vi "Convert_ERDS_GEA_Version.vi"(0 "New Header?":bool=TRUE, 2 "ERD Name":string[](array[string]), 5 "ERD_Data_Bound":T1, 7 "Multiple Read":T2 {"ERD Number" format="%x"}, 11 "error IO":errorcluster) -> (6 "All_ERD_Data_Bundled_Brass":T1, 15 "error out":errorcluster)   [LabVIEW 2021]
uses:
  Controles/Multiple_Read_ERD.ctl
  Controles/Read_ERD.ctl
  Controles/ERD_Data_Boundled.ctl
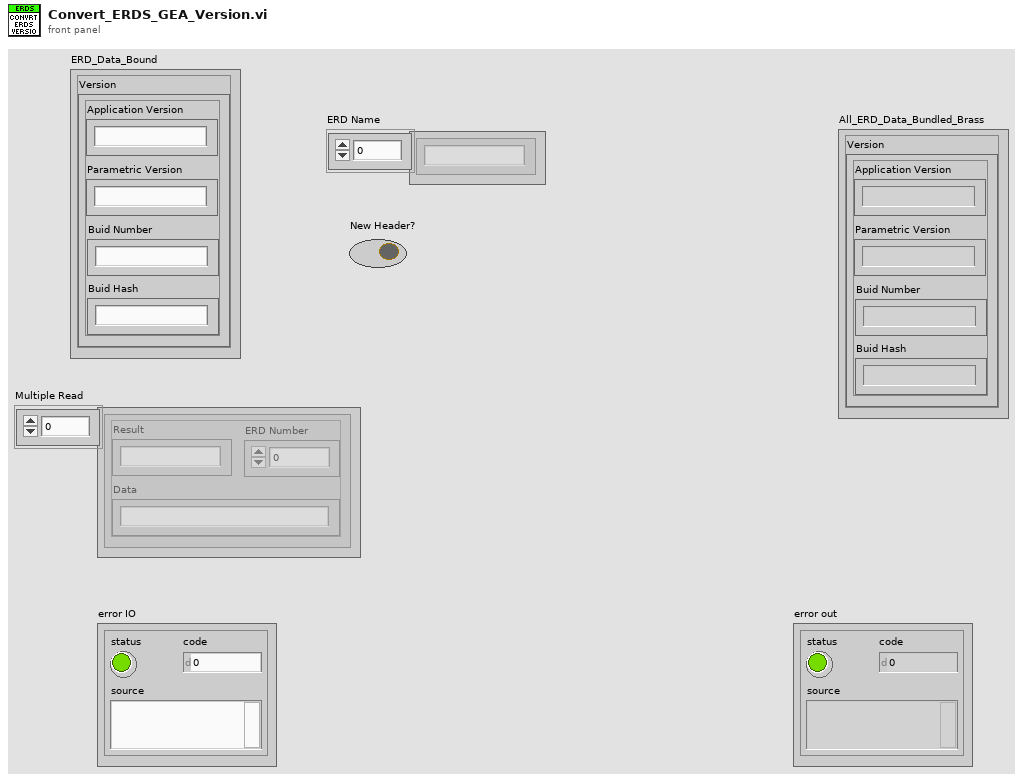
[diagram p1: front panel]
types:
  T1 = typedef "ERD_Data_Boundled.ctl" = cluster{"Version":cluster{"Application Version":string, "Parametric Version":string, "Buid Number":string, "Buid Hash":string}}
  T2 = typedef "Multiple_Read_ERD.ctl" = T3[]
  T3 = typedef "Read_ERD.ctl" = cluster{"Result":string, "ERD Number":i64, "Data":string}
  T4 = cluster{"Application Version":string, "Parametric Version":string, "Buid Number":string, "Buid Hash":string}
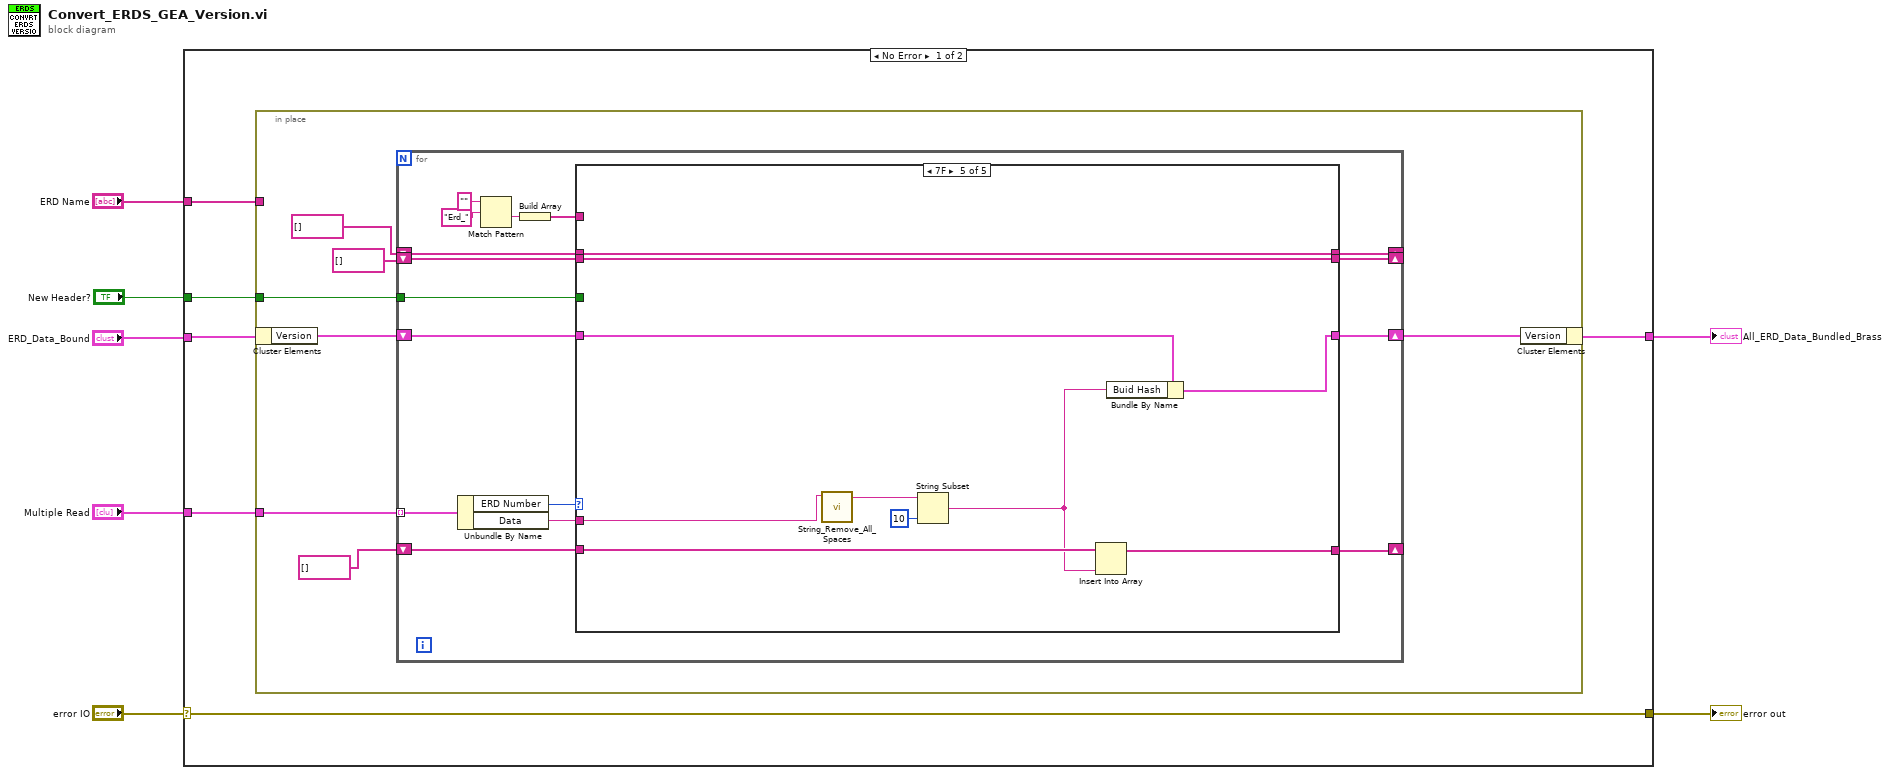
[diagram p0: block diagram]
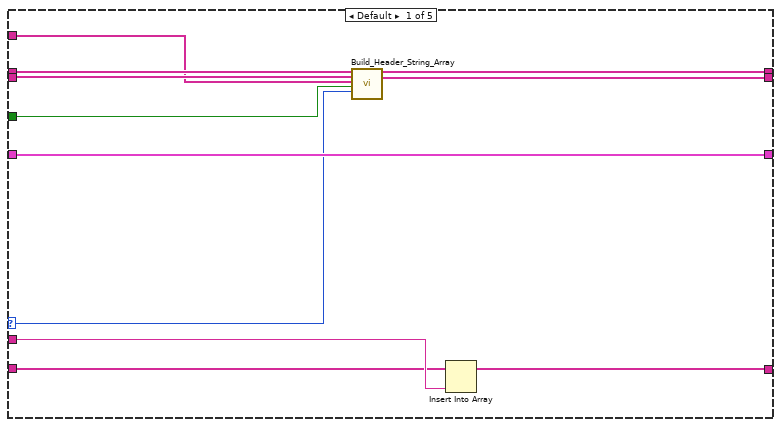
[diagram p2: hidden frame]
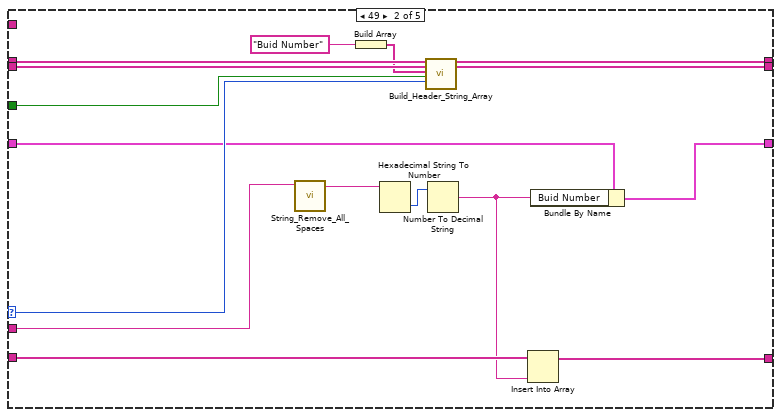
[diagram p3: hidden frame]
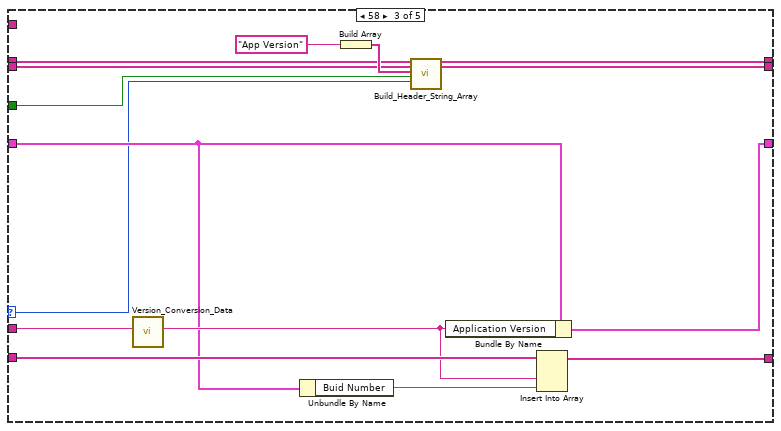
[diagram p4: hidden frame]
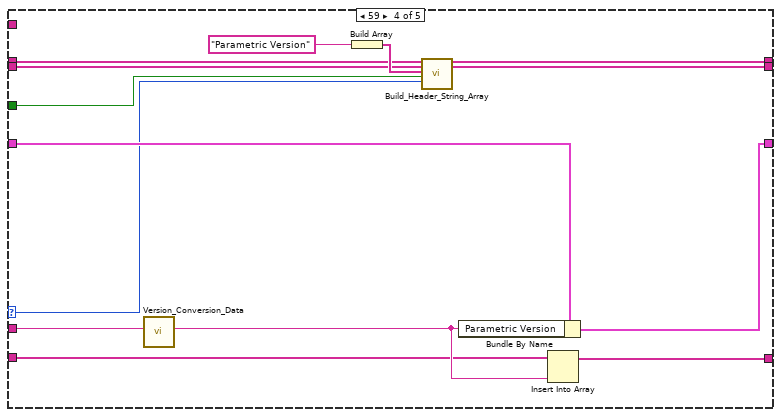
[diagram p5: hidden frame]
diagram:
  n1 = case shown="No Error" "error IO" {
    selector: "error IO" -> [w9 w103]
    tunnel: "ERD_Data_Bound" -> [w13 _]
    tunnel: "Multiple Read" -> [w12 _]
    tunnel: "ERD Name" -> [w11 _]
    tunnel: "New Header?" -> [w10 _]
    tunnel: [w9 w103] -> w2
    tunnel: [w8 _] -> w1
    frame No Error {
      n2 = in-place {
        in-place-border: w12 -> [w20]
        in-place-border: w11 -> [_]
        in-place-border: w10 -> [w15]
        n3 = in-place-cluster #1(w13) -> ("Version"=w17:T4)
        n4 = for {
          tunnel: w20 -> [w36] mode=indexing
          shift-right: [w31] -> _
          shift-left: string[] [] ("ERD Name Array Out") -> [w30]
          shift-right: [w29] -> _
          shift-left: string[] [] ("ERD Number Array Out") -> [w28]
          shift-right: [w26] -> _
          shift-left: string[] [] ("ERD String Data") -> [w25]
          shift-right: [w23] -> w16
          shift-left: w17 -> [w24]
          tunnel: w15 -> [w22]
          n5 = Unbundle By Name(w36) -> ("ERD Number"=w35:i64, "Data"=w27:string)
          n6 = Match Pattern(string="", regular expression="Erd_") -> (after substring=w33:string)  [unwired: 1 in, 3 out]
          n7 = Build Array(w33) -> (w32:string[])
          n8 = case shown="7F" w35 {
            selector: w35 -> [w44 w57 w65 w80 _]
            tunnel: w32 -> [w42 _ _ _ _]
            tunnel: [w41 w63 w67 w83 w100] -> w31
            tunnel: w30 -> [w46 w62 w69 w85 w100]
            tunnel: [w40 w61 w66 w82 w99] -> w29
            tunnel: w28 -> [w45 w60 w68 w84 w99]
            tunnel: w27 -> [w39 w56 w76 w89 w102]
            tunnel: [w37 w53 w77 w87 w93] -> w26
            tunnel: w25 -> [w38 w52 w78 w88 w101]
            tunnel: w24 -> [w47 w51 w73 w81 w95]
            tunnel: [w47 w49 w74 w86 w94] -> w23
            tunnel: w22 -> [w43 w48 w64 w79 _]
            frame Default {
              n9 = call "Build_Header_String_Array.vi"("ERD Name Array In"=w46, "ERD Number Array In"=w45, "ERD Name List"=w42, "New Header?"=w43, "ERD Number"=w44) -> ("ERD Name Array Out"=w41:string[], "ERD Number Array Out"=w40:string[])  [unwired: 13 in]
              n10 = Insert Into Array(array=w38, new element=w39) -> (w37:string[])  [unwired: 1 in]
            }
            frame 49 {
              n11 = call "String_Remove_All_Spaces.vi"("input string"=w56) -> ("result string"=w54:string)  [unwired: 10 in]
              n12 = Build Array("Buid Number") -> (w59:string[])
              n13 = Hexadecimal String To Number(string=w54) -> (number=w55:u32)  [unwired: 2 in, 1 out]
              n14 = call "Build_Header_String_Array.vi"("ERD Name Array In"=w62, "ERD Number Array In"=w60, "ERD Name List"=w59, "New Header?"=w48, "ERD Number"=w57) -> ("ERD Name Array Out"=w63:string[], "ERD Number Array Out"=w61:string[])  [unwired: 13 in]
              n15 = Number To Decimal String(number=w55) -> (decimal integer string=w50:string)  [unwired: 1 in]
              n16 = Insert Into Array(array=w52, new element=w50) -> (w53:string[])  [unwired: 1 in]
              n17 = Bundle By Name(cluster=w51, "Buid Number"=w50) -> (w49:T4)
            }
            frame 58 {
              n18 = call "Version_Conversion_Data.vi"("Version In"=w76) -> ("Version Out"=w75:string)  [unwired: 9 in, 1 out]
              n19 = Unbundle By Name(w73) -> ("Buid Number"=w72:string)
              n20 = Build Array("App Version") -> (w71:string[])
              n21 = call "Build_Header_String_Array.vi"("ERD Name Array In"=w69, "ERD Number Array In"=w68, "ERD Name List"=w71, "New Header?"=w64, "ERD Number"=w65) -> ("ERD Name Array Out"=w67:string[], "ERD Number Array Out"=w66:string[])  [unwired: 13 in]
              n22 = Bundle By Name(cluster=w73, "Application Version"=w75) -> (w74:T4)
              n23 = Insert Into Array(array=w78, new element #1=w75, new element #2=w72) -> (w77:string[])  [unwired: 1 in]
            }
            frame 59 {
              n24 = call "Version_Conversion_Data.vi"("Version In"=w89) -> ("Version Out"=w92:string)  [unwired: 9 in, 1 out]
              n25 = Build Array("Parametric Version") -> (w91:string[])
              n26 = call "Build_Header_String_Array.vi"("ERD Name Array In"=w85, "ERD Number Array In"=w84, "ERD Name List"=w91, "New Header?"=w79, "ERD Number"=w80) -> ("ERD Name Array Out"=w83:string[], "ERD Number Array Out"=w82:string[])  [unwired: 13 in]
              n27 = Bundle By Name(cluster=w81, "Parametric Version"=w92) -> (w86:T4)
              n28 = Insert Into Array(array=w88, new element=w92) -> (w87:string[])  [unwired: 1 in]
            }
            frame 127 {
              n29 = call "String_Remove_All_Spaces.vi"("input string"=w102) -> ("result string"=w98:string)  [unwired: 10 in]
              n30 = String Subset(string=w98, length (rest)=10 ("length (rest)")) -> (substring=w96:string)  [unwired: 1 in]
              n31 = Insert Into Array(array=w101, new element=w96) -> (w93:string[])  [unwired: 1 in]
              n32 = Bundle By Name(cluster=w95, "Buid Hash"=w96) -> (w94:T4)
            }
          }
        }
        n33 = in-place-cluster #1("Version"=w16) -> (w8:T1)
      }
    }
    frame Error {
    }
  }
  "error out" <- w2
  "All_ERD_Data_Bundled_Brass" <- w1
